vi "Set Key Value (Single).vi"(5 "Key name":string, 6 "Key value":sgl, 7 "Section name":string, 8 "error in (no error)":errorcluster, 9 "Create key? [T]":bool=TRUE, 10 "Create section? [T]":bool=TRUE, 11 "Carya Config in":refnum<class "Carya Config.lvclass">) -> (0 "error out":errorcluster, 1 "Created key?":bool, 2 "Created session?":bool, 3 "Carya Config out":refnum<class "Carya Config.lvclass">, 4 "Value written?":bool)   [LabVIEW 2013, in "Carya Config.lvclass"]
doc: "Copyright 2018, Carya Automatisering, Wiebe Walstra."
uses:
  Carya Config.lvclass
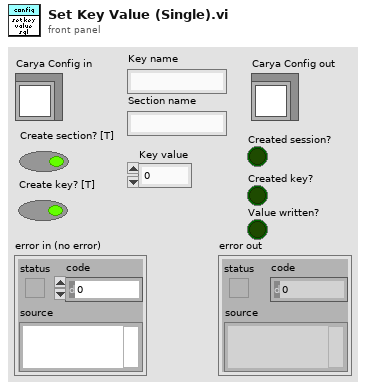
[diagram p1: front panel]
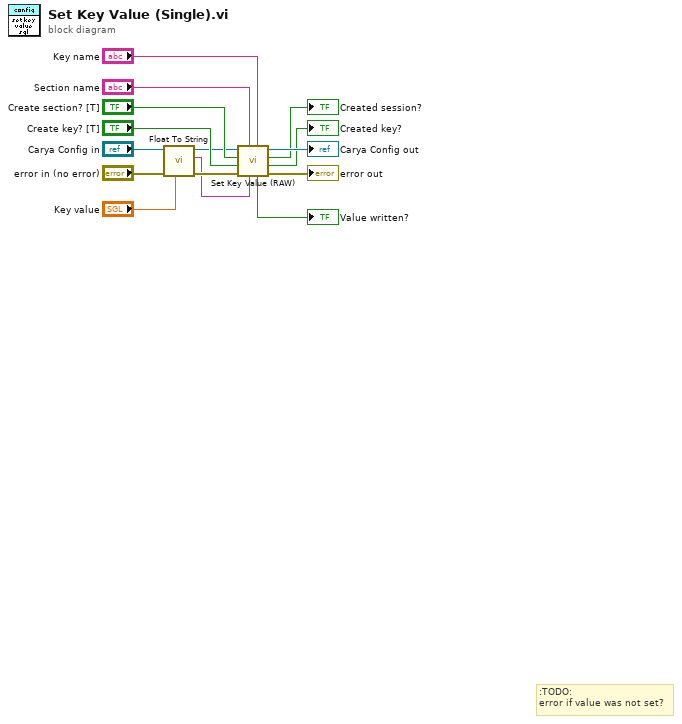
[diagram p0: block diagram]
diagram:
  # ":TODO:\nerror if value was not set?"
  n1 = call-dynamic "Float To String.vi"("Variant"="Key value", "error in (no error)"="error in (no error)", "Registry Object"="Carya Config in") -> ("error out"=w5:errorcluster, "resulting string"=w1:string, "Registry Object"=w3:refnum<class "Carya Config.lvclass">)  [unwired: 6 in]
  n2 = call-dynamic "Set Key Value (RAW).vi"("Key name"="Key name", "Key value"=w1, "Section name"="Section name", "error in (no error)"=w5, "Create key? [T]"="Create key? [T]", "Create section? [T]"="Create section? [T]", "Carya Config in"=w3) -> ("error out"=→"error out":errorcluster, "Created key?"=→"Created key?":bool, "Created session?"=→"Created session?":bool, "Carya Config out"=→"Carya Config out":refnum<class "Carya Config.lvclass">, "Value written?"=→"Value written?":bool)
